vi "Power_spectrum_Autocorrelation.vi"(5 "CompositeArrayIn":dbl[](array[numeric]) format="%.2f", 6 "Time (s)":dbl[](array[numeric]), 7 "Time Trace":T2, 8 "AnalysisInfoIn":T3={"Colour"=0, "Inst type"=enum."Pitot-static tube", "Inst name"="Manometer voltage", "Symbol"="U", "Code name"="", "Extra Info"="U", "Inst Array"=enum."PWA", "U"=0.0, "u^2"=0.0, "u^3"=0.0, "u^4"=0.0, "Skew_u"=0.0, "Kurt_u"=0.0, "Sd Error in Mean"=0.0, "% u'/U"=0.0, "X"=0.0, "Y"=0.0, "Z"=0.0, "Timescale integral Estimate"=0.0, "Sd Error in Variance"=0.0, "Calib File"=path "", "Calib Constants"=[], "Output Position"=FALSE, "Stats"=enum."None", "Av Sampling Rate"=0.0, "Av No of Samples"=0.0, "Total Meas Time (s)"=0.0, "OrigChName"="", "Max value"=0.0, "Min value"=0.0, "Req Sample Rate Hz"=0.0, "Sync Delay Time (s)"=0.0, "Ch No"=0, "Device"="", "Use Latest Calib"=FALSE, "Port"="", "Metadata Ch Names"=[], "Metadata Ch Values"=[], "Label"="", "chState"=enum."Solo", "Point Drift"=0.0, "inputConfig"=""} {"Kurt_u" format="%_3g"; "u^4" format="%_3g"; "u^3" format="%_3g"; "Sd Error in Variance" format="%_3g"; "u^2" format="%_3g"; "Sd Error in Mean" format="%_3g"; "U" format="%_3g"; "Sync Delay Time (s)" format="%.4f"; "Total Meas Time (s)" format="%_5g"; "Skew_u" format="%_3g"; "% u'/U" format="%_3g"}) -> (0 "CompositeArrayOut":dbl[](array[numeric]) format="%.2f", 1 "Autocorrelation":T1 {"X array" format="%^_5g"; "Y array" format="%^_5g"}, 2 "Spectra":T1 {"X array" format="%^_5g"; "Y array" format="%^_5g"}, 3 "AnalysisInfoOut":T3={"Colour"=0, "Inst type"=enum."Pitot-static tube", "Inst name"="Manometer voltage", "Symbol"="U", "Code name"="", "Extra Info"="U", "Inst Array"=enum."PWA", "U"=0.0, "u^2"=0.0, "u^3"=0.0, "u^4"=0.0, "Skew_u"=0.0, "Kurt_u"=0.0, "Sd Error in Mean"=0.0, "% u'/U"=0.0, "X"=0.0, "Y"=0.0, "Z"=0.0, "Timescale integral Estimate"=0.0, "Sd Error in Variance"=0.0, "Calib File"=path "", "Calib Constants"=[], "Output Position"=FALSE, "Stats"=enum."None", "Av Sampling Rate"=0.0, "Av No of Samples"=0.0, "Total Meas Time (s)"=0.0, "OrigChName"="", "Max value"=0.0, "Min value"=0.0, "Req Sample Rate Hz"=0.0, "Sync Delay Time (s)"=0.0, "Ch No"=0, "Device"="", "Use Latest Calib"=FALSE, "Port"="", "Metadata Ch Names"=[], "Metadata Ch Values"=[], "Label"="", "chState"=enum."Solo", "Point Drift"=0.0, "inputConfig"=""} {"Kurt_u" format="%_3g"; "u^4" format="%_3g"; "u^3" format="%_3g"; "Sd Error in Variance" format="%_3g"; "u^2" format="%_3g"; "Sd Error in Mean" format="%_3g"; "U" format="%_3g"; "Sync Delay Time (s)" format="%.4f"; "Total Meas Time (s)" format="%_5g"; "Skew_u" format="%_3g"; "% u'/U" format="%_3g"})   [LabVIEW 2022 SP3]
uses:
  Globals/Meas_global.vi
  Controls/XY_Plot_Cluster.ctl
  Controls/Inst_type.ctl
  Controls/Instrument_Array.ctl
  Controls/Analysis_info_cluster.ctl
  Controls/Time_Trace_Cluster.ctl
  Controls/channelState.ctl
panel:
  out "No of Resampled samples":dbl format="%_6g"
  out "size(s)":i32
  out "Spectrum":cluster{dbl[], dbl[]}(graph)
  # "Contains SamplingFrequency, nSamples, \nSpectrum, then Autocorrelation, all in one array..."
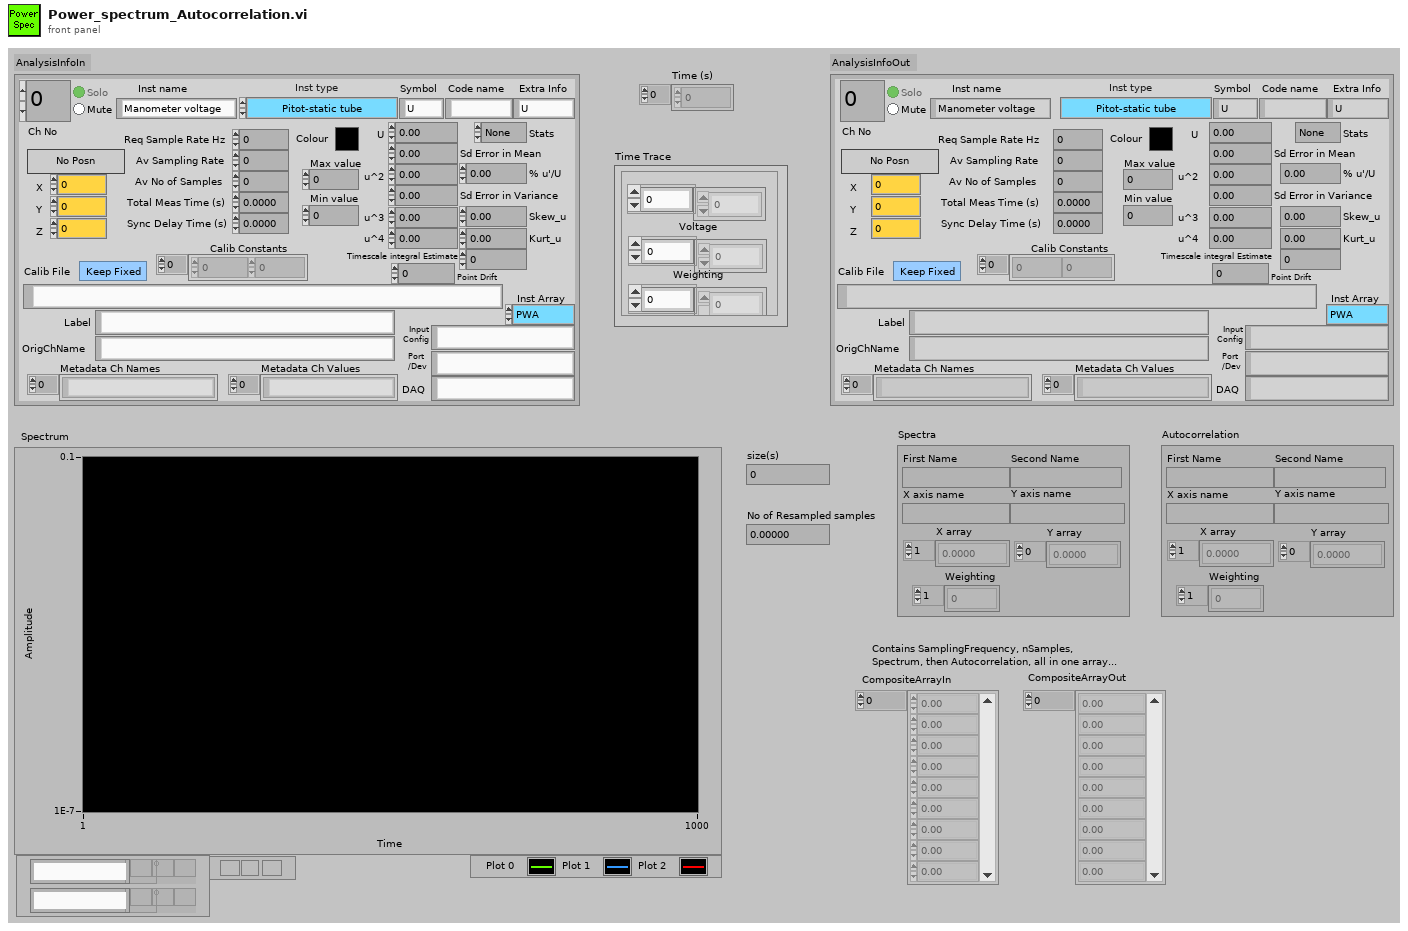
[diagram p1: front panel]
types:
  T1 = typedef "XY_Plot_Cluster.ctl" = cluster{"First Name":string, "Second Name":string, "X axis name":string, "Y axis name":string, "X array":dbl[], "Y array":dbl[], "Weighting":dbl[]}
  T2 = typedef "Time_Trace_Cluster.ctl" = cluster{"Weighting":dbl[], "Voltage":dbl[], "Eng Values":dbl[]}
  T3 = typedef "Analysis_info_cluster.ctl" = cluster{"Colour":u32, "Inst type":T4, "Inst name":string, "Symbol":string, "Code name":string, "Extra Info":string, "Inst Array":T5, "U":dbl, "u^2":dbl, "u^3":dbl, "u^4":dbl, "Skew_u":dbl, "Kurt_u":dbl, "Sd Error in Mean":dbl, "% u'/U":dbl, "X":dbl, "Y":dbl, "Z":dbl, "Timescale integral Estimate":dbl, "Sd Error in Variance":dbl, "Calib File":path, "Calib Constants":dbl[], "Output Position":bool, "Stats":enum16{"None", "Basic", "Full"}, "Av Sampling Rate":dbl, "Av No of Samples":dbl, "Total Meas Time (s)":dbl, "OrigChName":string, "Max value":dbl, "Min value":dbl, "Req Sample Rate Hz":dbl, "Sync Delay Time (s)":dbl, "Ch No":i16, "Device":string, "Use Latest Calib":bool, "Port":string, "Metadata Ch Names":string[], "Metadata Ch Values":string[], "Label":string, "chState":T6, "Point Drift":dbl, "inputConfig":string}
  T4 = typedef "Inst_type.ctl" = enum16{"Raw voltage", "Raw with zero offsetting", "Propeller anemometer", "Pressure Transducer", "Pitot-static tube", "Hot wire", "Cross wire 1", "Cross wire 2", "Generic Linear", "Generic Polynomial", "Generic BackPoly", "Fast FID", "Thermocouple", "Cold wire", "Pulsed Wire", "LDA Vel", "LDA Tran time", "LDA Arr time", "Microphone"}
  T5 = typedef "Instrument_Array.ctl" = enum16{"PWA", "LDA", "Analogue"}
  T6 = typedef "channelState.ctl" = enum32{"No Selection", "Solo", "Mute"}
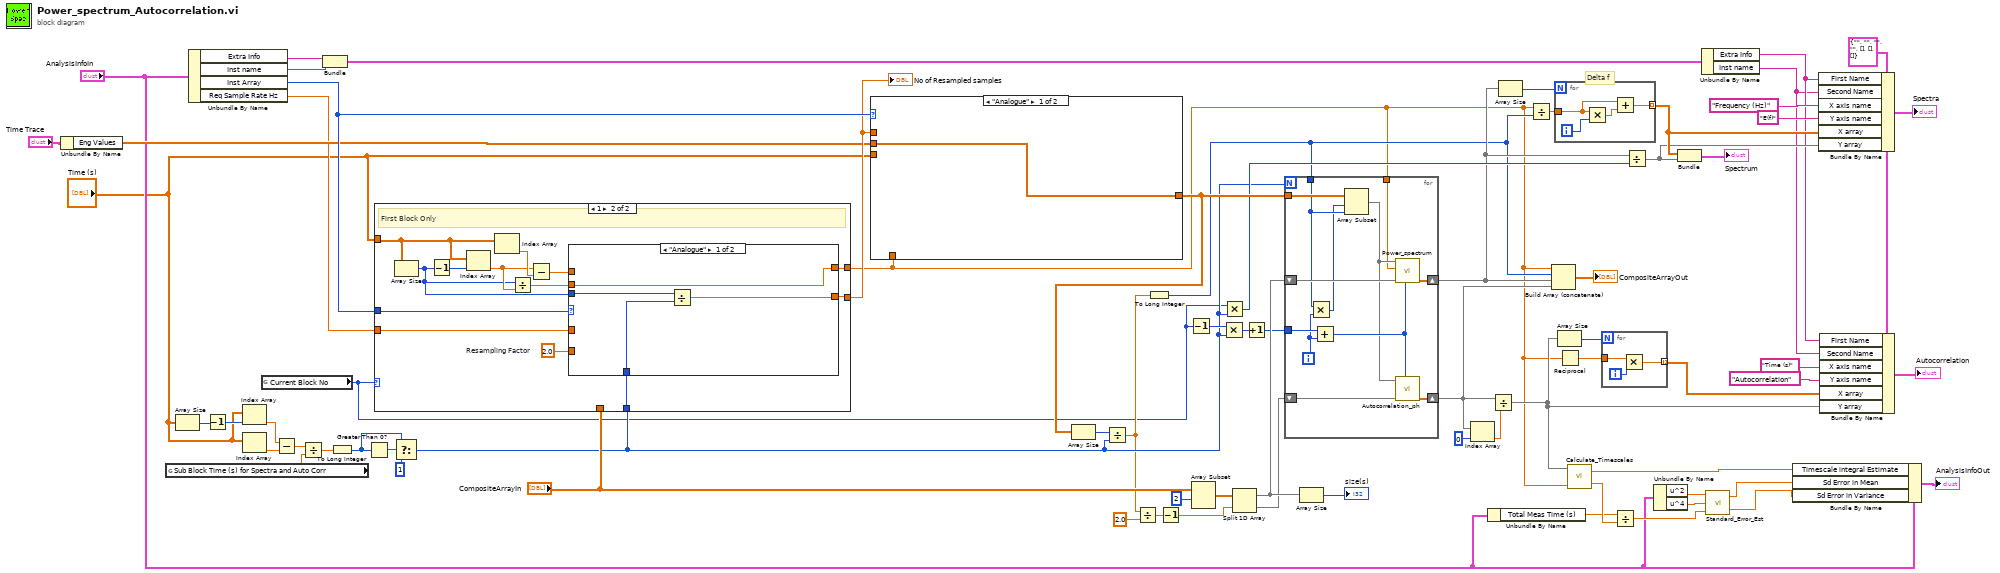
[diagram p0: block diagram]
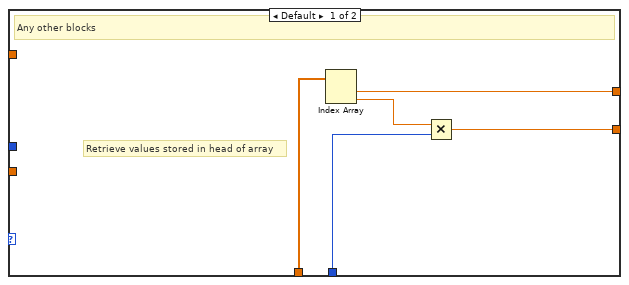
[diagram p2: hidden frame]
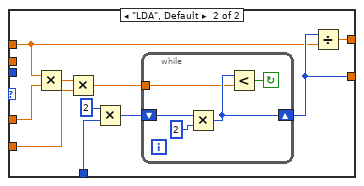
[diagram p3: hidden frame]
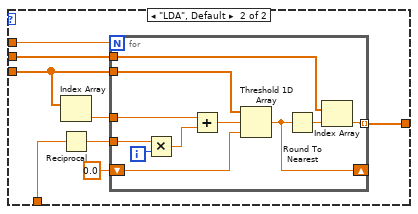
[diagram p4: hidden frame]
diagram:
  w8 = T1 {"First Name"="", "Second Name"="", "X axis name"="", "Y axis name"="", "X array"=[], "Y array"=[], "Weighting"=[]} ("element")
  # "Delta f"
  n1 = Unbundle By Name("Time Trace") -> ("Eng Values"=w36:dbl[])
  n2 = global read "Meas_global.vi" "Sub Block Time (s) for Spectra and Auto Corr"() -> (w22:dbl)
  n3 = Array Size(array="Time (s)") -> (size(s)=w26:i32)
  n4 = Unbundle By Name("AnalysisInfoIn") -> ("Extra Info"=w66:string, "Inst name"=w64:string, "Inst Array"=w70:T5, "Req Sample Rate Hz"=w28:dbl)
  n5 = Decrement(x=w26) -> (x-1=w27:i32)
  n6 = Index Array(array="Time (s)", index=w27) -> (element=w24:dbl)
  n7 = Index Array(array="Time (s)") -> (element=w25:dbl)  [unwired: 1 in]
  n8 = global read "Meas_global.vi" "Current Block No"() -> (w5:i32)
  n9 = Subtract(x=w24, y=w25) -> (x-y=w23:dbl)
  n10 = Divide(x=w23, y=w22) -> (x/y=w21:dbl)
  n11 = Bundle("Extra Info"=w66, "Inst name"=w64) -> (w65:cluster{"Extra Info":string, "Inst name":string})  [unwired: 1 in]
  n12 = To Long Integer(number=w21) -> (32bit integer=w19:i32)
  n13 = Greater Than 0?(x=w19) -> (x > 0?=w20:bool)
  n14 = Select(t=w19, s=w20, f=1) -> (s? t:f=w16:i32)
  n15 = case shown="1" w5 {
    tunnel: "Time (s)" -> [_ w85]
    tunnel: [w76 w88] -> w2
    tunnel: "CompositeArrayIn" -> [w77 _]
    tunnel: w70 -> [_ w89]
    tunnel: [w73 w87] -> w56
    tunnel: w16 -> [w74 w81]
    tunnel: w28 -> [_ w80]
    frame Default {
      # "Retrieve values stored in head of array"
      # "Any other blocks"
      n16 = Index Array(array=w77) -> (element #1=w76:dbl, element #2=w75:dbl)  [unwired: 2 in]
      n17 = Multiply(x=w75, y=w74) -> (x*y=w73:dbl)
    }
    frame 1 {
      w86 = 2.0  # Resampling Factor
      # "First Block Only"
      n18 = Array Size(array=w85) -> (size(s)=w78:i32)
      n19 = Decrement(x=w78) -> (x-1=w79:i32)
      n20 = Index Array(array=w85, index=w79) -> (element=w82:dbl)
      n21 = Index Array(array=w85) -> (element=w84:dbl)  [unwired: 1 in]
      n22 = Divide(x=w78, y=w82) -> (x/y=w90:dbl)
      n23 = Subtract(x=w82, y=w84) -> (x-y=w83:dbl)
      n24 = case shown="\"Analogue\"" w89 {
        tunnel: w90 -> [w94 _]
        tunnel: w83 -> [_ w97]
        tunnel: [w94 w104] -> w88
        tunnel: w78 -> [w93 _]
        tunnel: [w91 w102] -> w87
        tunnel: w86 -> [_ w101]
        tunnel: w81 -> [w92 w99]
        tunnel: w80 -> [_ w96]
        frame "Analogue" {
          n25 = Divide(x=w93, y=w92) -> (x/y=w91:dbl)
        }
        frame "LDA", Default {
          n26 = Multiply(x=w97, y=w96) -> (x*y=w95:dbl)
          n27 = Multiply(x=w95, y=w101) -> (x*y=w103:dbl)
          n28 = Multiply(x=2, y=w99) -> (x*y=w98:i32)
          n29 = while {
            shift-right: [w107] -> w102
            shift-left: w98 -> [w109]
            tunnel: w103 -> [w105]
            stop <- w106 continue-if-true
            n30 = Multiply(x=w109, y=2) -> (x*y=w107:i32)
            n31 = Less?(x=w107, y=w105) -> (x < y?=w106:bool)
          }
          n32 = Divide(x=w102, y=w97) -> (x/y=w104:dbl)
        }
      }
    }
  }
  "No of Resampled samples" <- w56
  n33 = case shown="\"Analogue\"" w70 {
    tunnel: w36 -> [w110 w112]
    tunnel: "Time (s)" -> [_ w114]
    tunnel: [w110 w111] -> w31
    tunnel: w56 -> [_ w118]
    tunnel: w2 -> [_ w116]
    frame "Analogue" {
    }
    frame "LDA", Default {
      n34 = Index Array(array=w114) -> (element=w115:dbl)  [unwired: 1 in]
      n35 = Reciprocal(x=w116) -> (1/x=w117:dbl)
      n36 = for {
        N: w118 -> [_]
        tunnel: w117 -> [w129]
        tunnel: w115 -> [w127]
        tunnel: w114 -> [w125]
        shift-right: [w119] -> _
        shift-left: 0.0 -> [w123]
        tunnel: w112 -> [w121]
        tunnel: [w120] -> w111 mode=indexing
        i -> [w128]
        n37 = Multiply(x=w129, y=w128) -> (x*y=w126:dbl)
        n38 = Add(x=w127, y=w126) -> (x+y=w124:dbl)
        n39 = Threshold 1D Array(1:w123, 2:w124, 3:w125) -> (0:w119:dbl)
        n40 = Round To Nearest(number=w119) -> (nearest integer value=w122:dbl)
        n41 = Index Array(array=w121, index=w122) -> (element=w120:dbl)
      }
    }
  }
  n42 = Array Size(array=w31) -> (size(s)=w30:i32)
  n43 = Divide(x=w30, y=w16) -> (x/y=w10:dbl)
  n44 = Divide(x=w10, y=2.0) -> (x/y=w54:dbl)
  n45 = To Long Integer(number=w10) -> (32bit integer=w9:i32)
  n46 = Decrement(x=w54) -> (x-1=w11:dbl)
  n47 = Decrement(x=w5) -> (x-1=w17:i32)
  n48 = Array Subset(array="CompositeArrayIn", index=2) -> (w57:dbl[])  [unwired: 1 in]
  n49 = Multiply(x=w17, y=w16) -> (x*y=w15:i32)
  n50 = Multiply(x=w5, y=w16) -> (x*y=w29:i32)
  n51 = Split 1D Array(array=w57, index=w11) -> (first subarray=w53:dbl[], second subarray=w52:dbl[])
  n52 = Increment(x=w15) -> (x+1=w14:i32)
  n53 = for {
    N: w16 -> [_]
    tunnel: w31 -> [w135]
    tunnel: w2 -> [w130]
    tunnel: w14 -> [w137]
    shift-right: [w138] -> w13
    shift-left: w52 -> [w139]
    shift-right: [w141] -> w12
    shift-left: w53 -> [w140]
    tunnel: w9 -> [w132]
    i -> [w133]
    n54 = Multiply(x=w132, y=w133) -> (x*y=w131:i32)
    n55 = Add(x=w137, y=w133) -> (x+y=w136:i32)
    n56 = Array Subset(array=w135, index=w131, length=w132) -> (w134:dbl[])
    n57 = call "Power_spectrum.vi"("Block No"=w136, "Spectrum input array"=w140, "Sampling frequency"=w130, "U"=w134) -> ("Spectrum Accumulator array"=w141:dbl[])  [unwired: 1 in, 3 out]
    n58 = call "Autocorrelation_ph.vi"("X"=w134, "Autocorrelation of X"=w139, "Block No"=w136) -> ("Autocorrelation of X"=w138:dbl[])  [unwired: 2 in, 1 out]
  }
  n59 = Array Size(array=w53) -> (size(s)=→"size(s)":i32)
  n60 = Index Array(array=w13, index=0 ("Index")) -> (element=w50:dbl)
  n61 = Unbundle By Name("AnalysisInfoIn") -> ("Total Meas Time (s)"=w3:dbl)
  n62 = Divide(x=w13, y=w50) -> (x/y=w45:dbl[])
  n63 = Array Size(array=w12) -> (size(s)=w68:i32)
  n64 = Divide(x=w2, y=w9) -> (x/y=w69:dbl)
  n65 = Build Array (concatenate)(w2, w9, w12, w13) -> (→"CompositeArrayOut":dbl[])
  n66 = for {
    N: w68 -> [_]
    tunnel: w69 -> [w142]
    tunnel: [w143] -> w61 mode=indexing
    i -> [w145]
    n67 = Multiply(x=w142, y=w145) -> (x*y=w144:dbl)
    n68 = Add(x=w142, y=w144) -> (x+y=w143:dbl)
  }
  n69 = Array Size(array=w45) -> (size(s)=w43:i32)
  n70 = Reciprocal(x=w2) -> (1/x=w47:dbl)
  n71 = call "Calculate_Timescales.vi"("Sampling Frequency (Hz)"=w2, "Autocorrelation"=w45) -> ("Time between independent samples (s)"=w32:dbl, "Timescale estimate (s)"=w33:dbl)  [unwired: 1 in]
  n72 = for {
    N: w43 -> [_]
    tunnel: w47 -> [w147]
    tunnel: [w146] -> w46 mode=indexing
    i -> [w148]
    n73 = Multiply(x=w147, y=w148) -> (x*y=w146:dbl)
  }
  n74 = Divide(x=w3, y=w32) -> (x/y=w40:dbl)
  n75 = Divide(x=w12, y=w29) -> (x/y=w60:dbl[])
  n76 = Unbundle By Name("AnalysisInfoIn") -> ("u^2"=w42:dbl, "u^4"=w41:dbl)
  n77 = Bundle(w61, w60) -> (→"Spectrum":cluster{dbl[], dbl[]})  [unwired: 1 in]
  n78 = Unbundle By Name(w65) -> ("Extra Info"=w7:string, "Inst name"=w6:string)
  n79 = call "Standard_Error_Est.vi"("N"=w40, "4th order moment u^4"=w41, "2nd order moment u^2"=w42) -> ("Standard error in variance"=w38:dbl, "Standard error in Mean"=w39:dbl)
  n80 = Bundle By Name(cluster="AnalysisInfoIn", "Timescale integral Estimate"=w33, "Sd Error in Mean"=w39, "Sd Error in Variance"=w38) -> (→"AnalysisInfoOut":T3)
  n81 = Bundle By Name(cluster=w8, "First Name"=w7, "Second Name"=w6, "X axis name"="Frequency (Hz)", "Y axis name"="E(f)", "X array"=w61, "Y array"=w60) -> (→"Spectra":T1)
  n82 = Bundle By Name(cluster=w8, "First Name"=w7, "Second Name"=w6, "X axis name"="Time (s)", "Y axis name"="Autocorrelation", "X array"=w46, "Y array"=w45) -> (→"Autocorrelation":T1)
